vi "STS_spectroscopy_V2.vi"(6 "Internal use":string, 7 "Grid param":T1 {"height (m)" format="%#_6p"; "width (m)" format="%#_6p"; "center Y (m)" format="%#_6p"; "center X (m)" format="%#_6p"}, 8 "Error in (no error)":errorcluster, 9 "Points Y/Index Y":i32, 10 "Points X/Index X":i32, 11 "Method":enum16{"init", "run", "end"}(ring)=enum."end") -> (0 "Error out":errorcluster)   [LabVIEW 2014]
doc: "Example of a measurement VI to be used in the \"Experiments on a Grid\" tool as external VI.\n\nThis example measure the topography and spectroscopy data. The spectroscopy measurements are taken on a subgrid. The data are saved to a sxm and a binary file.\n\n- Nanonis Programming Interface -"
uses:
  <userlib>/Nanonis Prog Interface V5/Scan/Grid/LinePatternGet.vi
  <userlib>/Nanonis Prog Interface V5/Scan/Grid/GridPatternGet.vi
  <userlib>/Nanonis Prog Interface V5/Scan/Grid/CloudPatternGet.vi
  <userlib>/Nanonis Prog Interface V5/Nanonis Prog Interface.lvlib
panel:
  in  "Ramp Bias On/Off":bool
  out "Status 2":string="finishing"
  in  "Lockin delay [ms]":u32
  in  "Z Controller ON/OFF":bool
  in  "type":u16(ring)=1 items=["Line", "Grid", "Cloud"]
  in  "Lockin ON/OFF":bool
  in  "Correct Drift":bool=TRUE
  in  "Email when finished":string="cornelius.krull@monash.edu, dhaneesh.gopalakrishnan@monash.edu"
  in  "STS z offset":dbl format="%#_6p"
  out "ETA":timestamp=timestamp(3582621546.85837 s since 1904-01-01)
  out "remaining":dbl=19834.093046092985 format="%<%H:%M:%S>t"
  out "Progress":u8(slide)=5 scale=0.0..100.0 scale format="%#.1g"
  out "total Points":i32=576
  in  "preSTS delay [ms]":u32=3
  in  "STS Bias":dbl=-3.4 format="%#_6p"
  in  "Move Bias":dbl=-3.4 format="%#_6p"
  in  "Move Current":dbl=5e-11 format="%#_6p"
  in  "Imaging Bias":dbl=-3.4 format="%#_6p"
  in  "max applied Drift Correction":i32=20 min=1 max=100 step=1 format="%.0p"
  in  "Correlate":u16(ring) items=["first Frame", "successive Frames"]
  out "Topo Images taken":i32
  in  "Increment":i32=40
  in  "Threshold":i32=2 min=1 step=1
  in  "tip Speed (m/s)":sgl=1e-08 format="%.2p"
  out "X drift":i32
  out "Y drift":i32
  out "Last Drift detected":i32
  in  "MaxImagesBack":i32=2
  in  "Channel index (0-23)":u8(ring) items=["Current"=0, "Z (m)"=14]
  in  "File name":string="DCA_cluster_STS_Grid"
  in  "STS Current":dbl=5e-11 format="%#_6p"
  in  "Imaging Current":dbl=5e-11 format="%#_6p"
  in  "zdrift \nDuration (s)":dbl
  in  "Correct z drift":bool
  out "Status":string="finishing"
  in  "Drift correction Pixels":i32=256 caption="Topo Pixels"
  out "Y Offset":dbl format="%#_6p"
  out "X Offset":dbl format="%#_6p"
  out "Points taken":dbl=30.0
  in  "Drift Correction every":i32=40
  in  "Y subgrid spacing":u16=1
  in  "X subgrid spacing":u16=1
  # "GRID points"
  # "Increase this if no Drift was detected for \na certain number of images"
  # "%"
  # "time (HH:MM:SS)"
  # "images back"
  # "% of image size"
  # "<--Z Cont. Needs to be off"
  # "RUN smart tilt before starting the GRID"
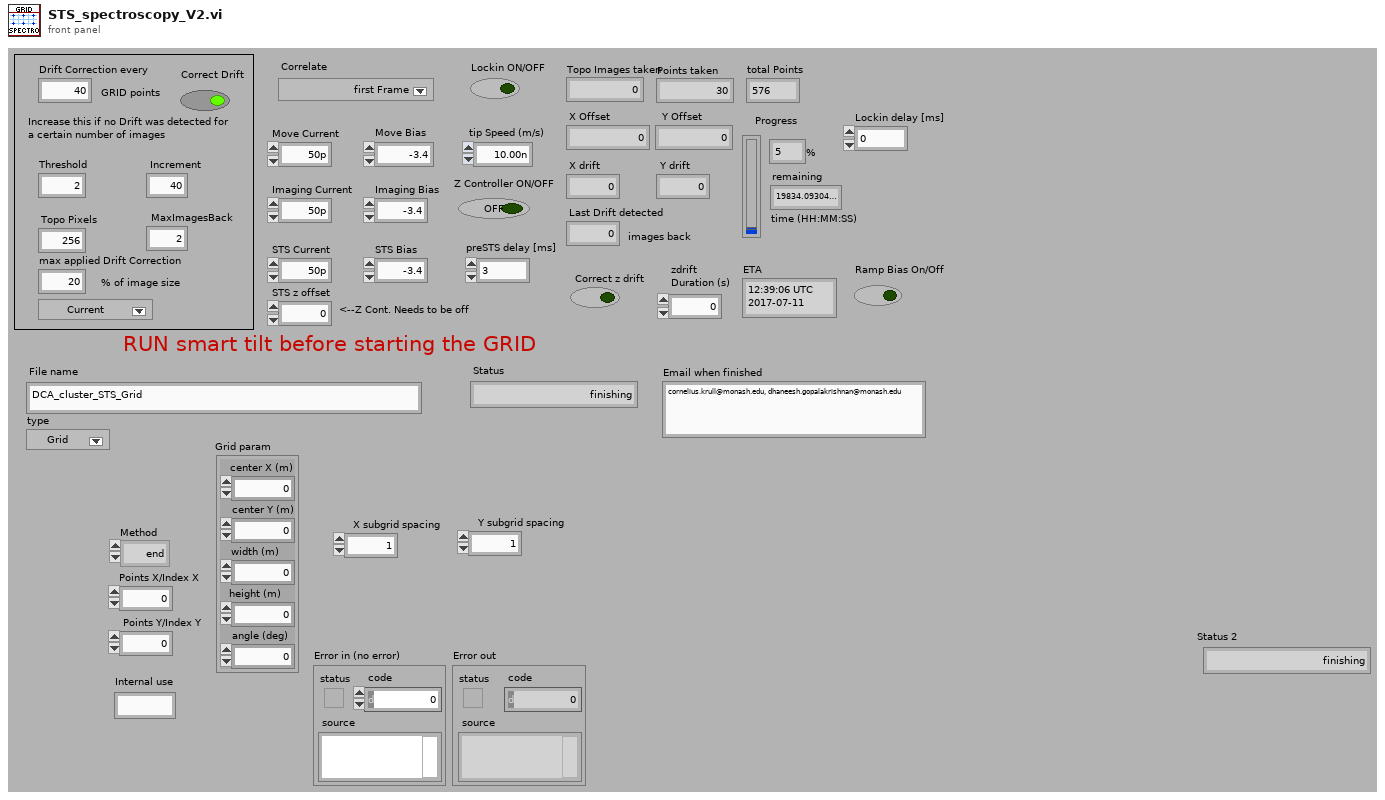
[diagram p1: front panel]
types:
  T1 = cluster{"center X (m)":sgl, "center Y (m)":sgl, "width (m)":sgl, "height (m)":sgl, "angle (deg)":sgl}
  T2 = cluster{"Drift correction Pixels":i32, "Imaging Current":dbl, "STS Current":dbl, "MaxImagesBack":i32, "tip Speed (m/s)":sgl, "Threshold":i32, "Increment":i32, "Correlate":u16, "max applied Drift Correction":i32, "Imaging Bias":dbl, "Move Current":dbl, "Move Bias":dbl, "STS Bias":dbl, "preSTS delay [ms]":u32, "STS z offset":dbl, "Correct Drift":bool, "Lockin ON/OFF":bool}
  T3 = cluster{"center X":sgl, "center Y":sgl, "angle":sgl, "width":sgl, "height":sgl, "# pixels":i32, "# lines":i32}
  T4 = cluster{"Name":string, "Calibration":sgl, "Offset":sgl, "Channel index":i32}[]
  T5 = cluster{"up/down":bool, "time/line":sgl, "start time":timestamp, "end time":timestamp}
  T6 = cluster{"Z averaging time (s)":sgl, "Z offset (m)":sgl, "Initial settling time (s)":sgl}
  T7 = cluster{"Max. slew rate (V/s)":sgl, "Settling time (s)":sgl, "Integration time (s)":sgl}
  T8 = cluster{"End settling time (s)":sgl, "Z control time (s)":sgl}
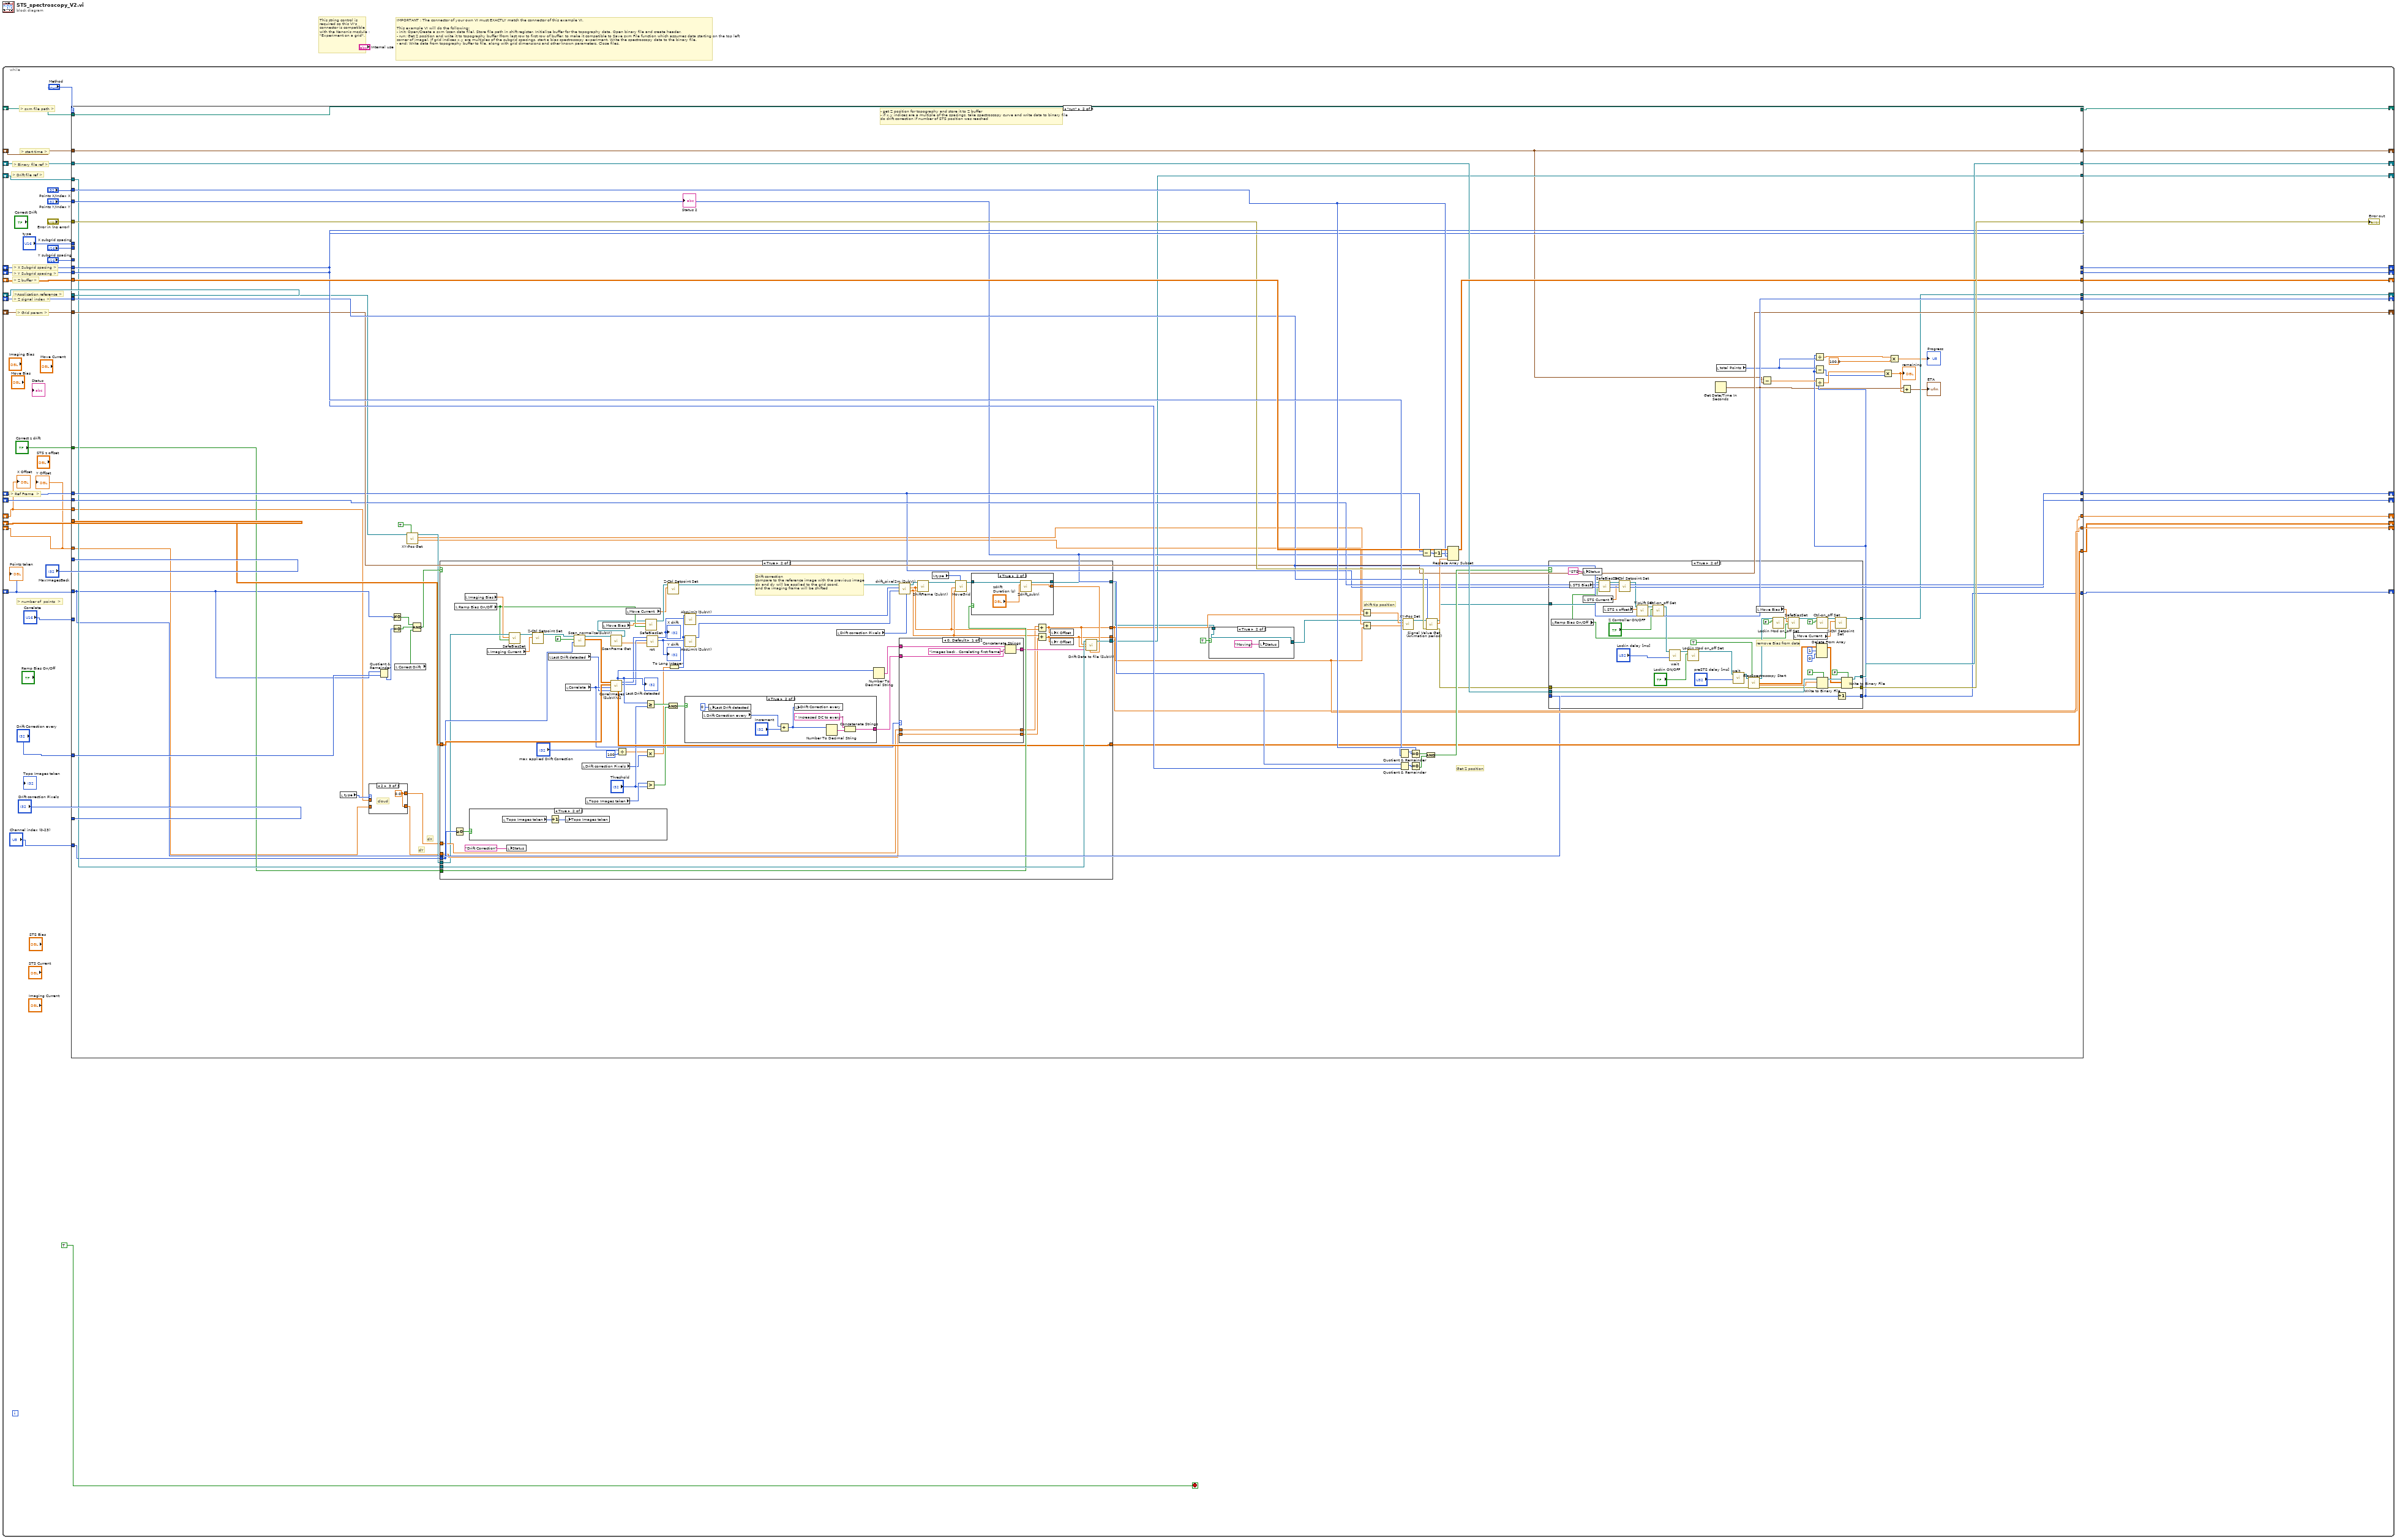
[diagram p0: block diagram]
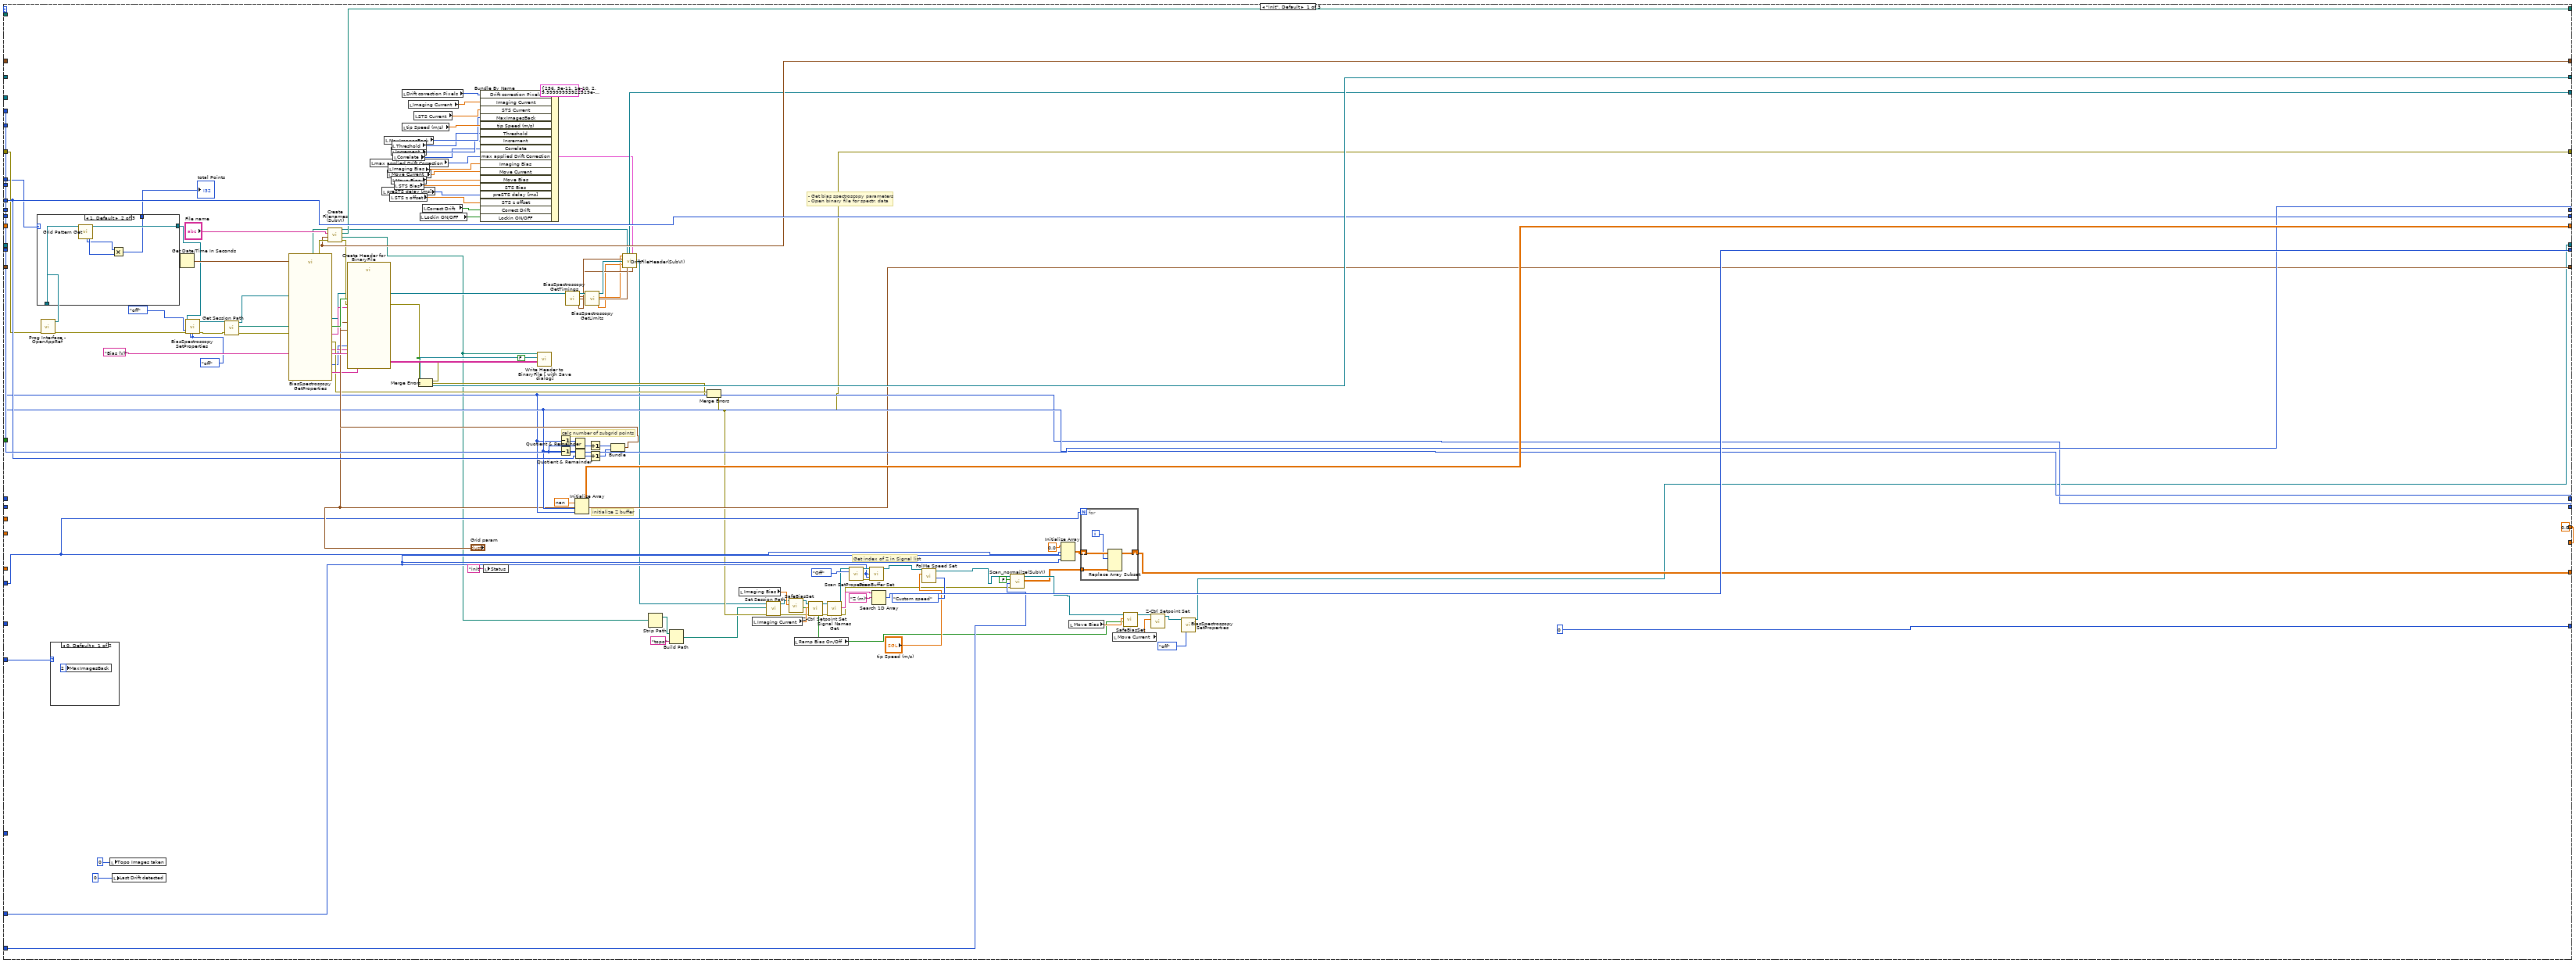
[diagram p2: hidden frame]
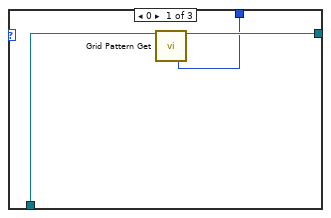
[diagram p3: hidden frame]
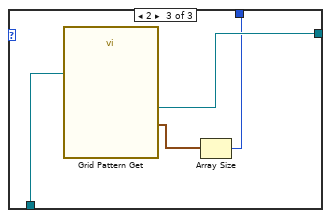
[diagram p4: hidden frame]
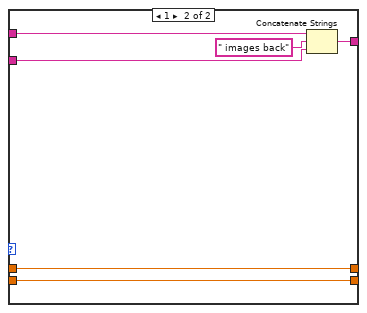
[diagram p10: hidden frame]
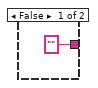
[diagram p12: hidden frame]
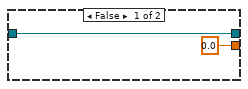
[diagram p13: hidden frame]
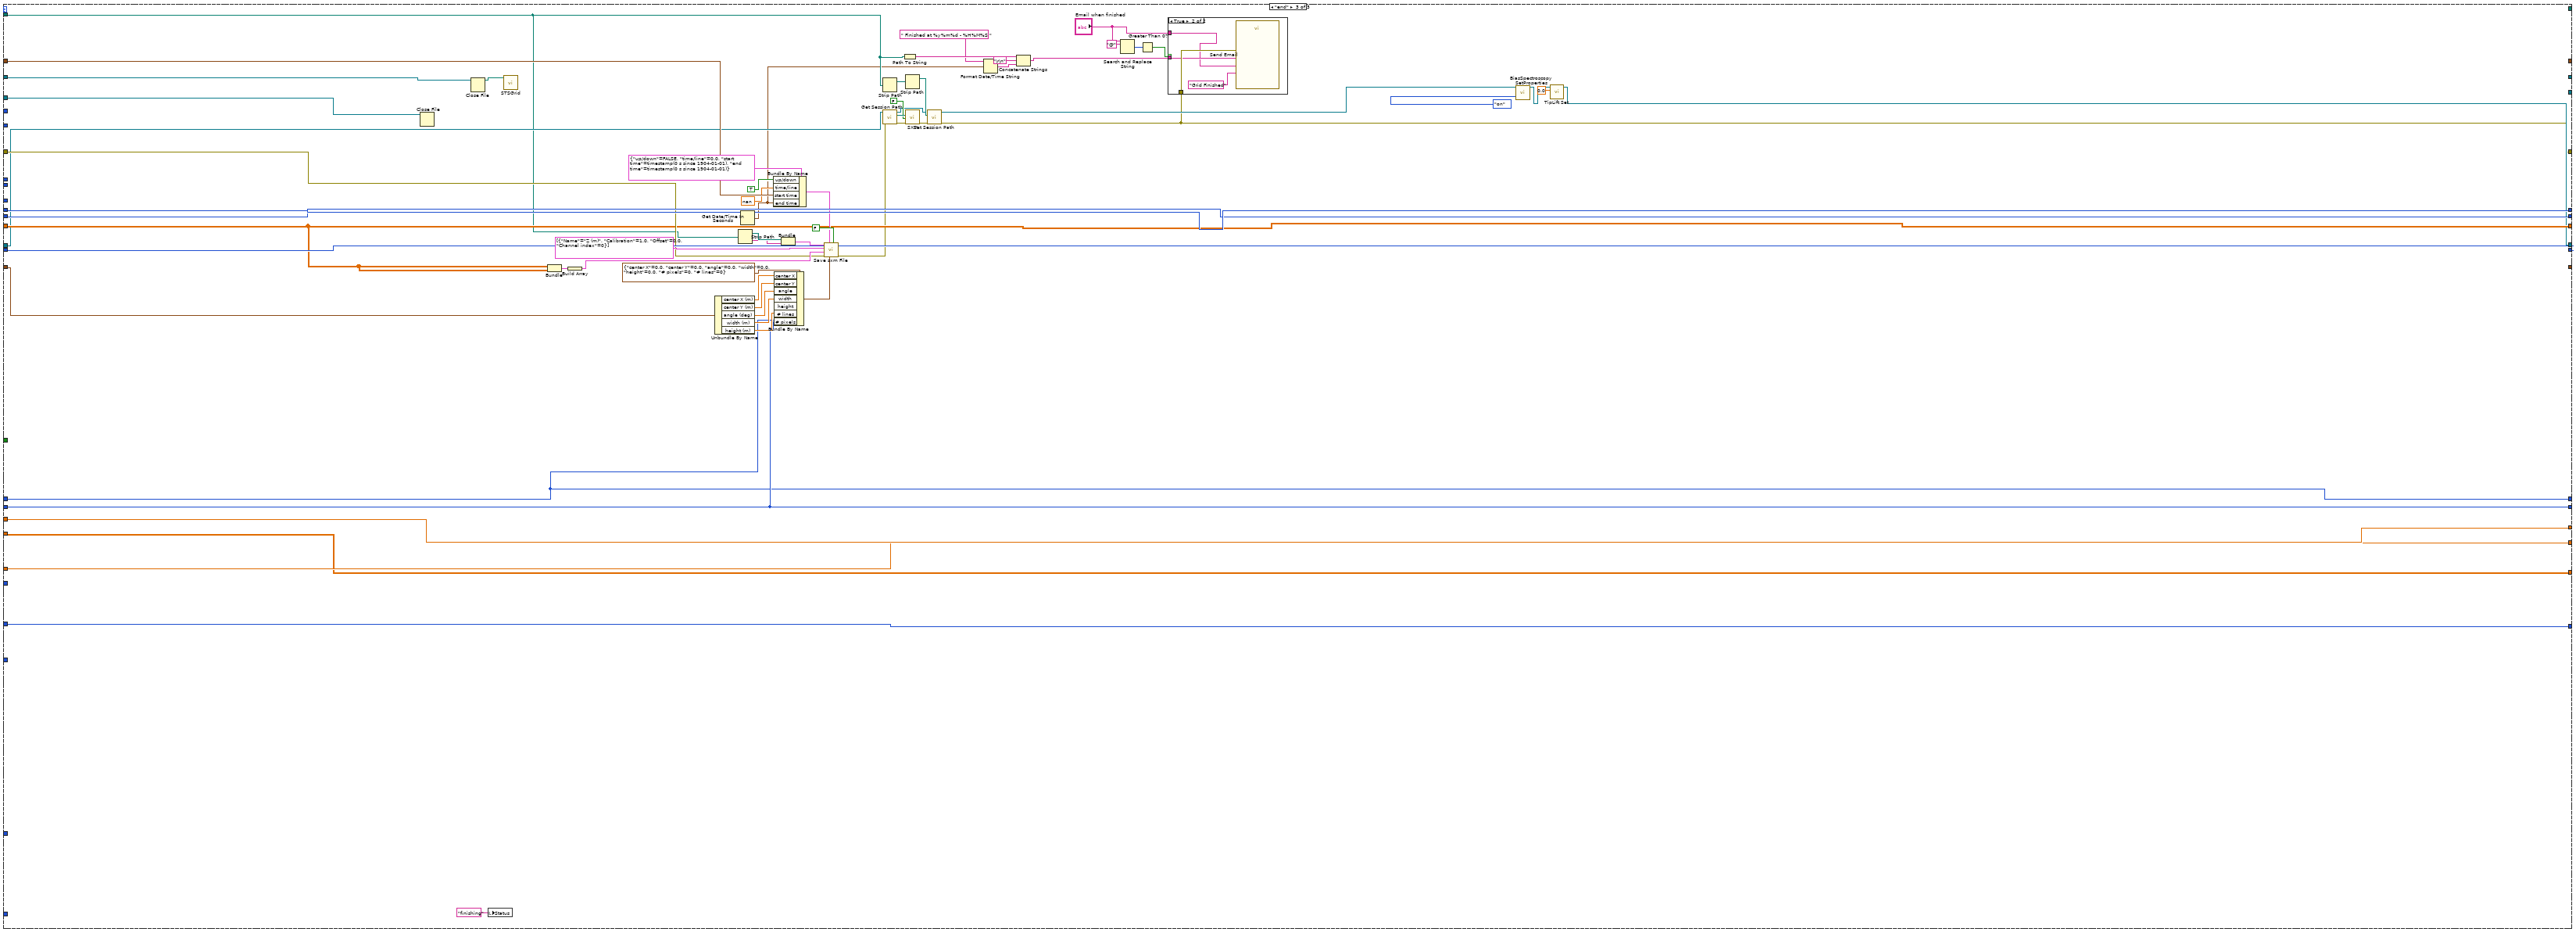
[diagram p15: hidden frame]
diagram:
  # "This string control is required so this VI's connector is compatible with the Nanonis module : \"Experiment on a grid\"."
  # "IMPORTANT : The connector of your own VI must EXACTLY match the connector of this example VI.\n\nThis example VI will do the following:\n- init: Open/Create a sxm (scan data file). Store file path in shift register. Initialize buffer for the topography data. Open binary file and create header.\n- run: Get Z position and write it to topography buffer (from last row to first row of buffer, to make it compatible to Save sxm File function which assumes data starting on the top left corner of image). If grid indices x,y are multiples of the subgrid spacings, start a bias spectroscopy experiment. Write the spectroscopy data to the binary file.\n- end: Write data from topography buffer to file, along with grid dimensions and other known parameters. Close files."
  n1 = while {
    shift-right: [w22] -> _
    shift-left: _ -> [w45]
    shift-right: [w40] -> _
    shift-left: _ -> [w39]
    shift-right: [w37] -> _
    shift-left: _ -> [w38]
    shift-right: [w36] -> _
    shift-left: _ -> [w35]
    shift-right: [w29] -> _
    shift-left: _ -> [w31]
    shift-right: [w30] -> _
    shift-left: _ -> [w32]
    shift-right: [w28] -> _
    shift-left: _ -> [w27]
    shift-right: [w26] -> _
    shift-left: _ -> [w25]
    shift-right: [w24] -> _
    shift-left: _ -> [w23]
    shift-right: [w21] -> _
    shift-left: _ -> [w20]
    shift-right: [w19] -> _
    shift-left: _ -> [w18]
    shift-right: [w17] -> _
    shift-left: _ -> [w10]
    shift-right: [w16] -> _
    shift-left: _ -> [w9]
    shift-right: [w15] -> _
    shift-left: _ -> [w12]
    shift-right: [w14] -> _
    shift-left: _ -> [w11]
    shift-right: [w7] -> _
    shift-left: _ -> [w6]
    stop <- TRUE stop-if-true
    # "> Drift file ref >"
    # "> number of  points  >"
    # "> Ref Frame  >"
    # "> Grid param >"
    # "> start time >"
    # ">Application reference >"
    # "> Y Subgrid spacing >"
    # "> X Subgrid spacing >"
    # "> Z signal index >"
    # "> Binary file ref >"
    # "> Z buffer >"
    # "> sxm file path >"
    n2 = case shown="\"run\"" "Method" {
      tunnel: [w128 w252 _] -> w22
      tunnel: w45 -> [_ w252 w421]
      tunnel: "Error in (no error)" -> [w130 w238 w448]
      tunnel: [w53 w251 w402] -> w43
      tunnel: "Points X/Index X" -> [w142 w246 _]
      tunnel: "Points Y/Index Y" -> [w143 w231 _]
      tunnel: [w166 w249 w437] -> w40
      tunnel: w39 -> [_ w250 w437]
      tunnel: w38 -> [_ w248 w430]
      tunnel: [w158 w247 _] -> w37
      tunnel: [w156 w236 w462] -> w36
      tunnel: w35 -> [_ w236 w462]
      tunnel: "X subgrid spacing" -> [w155 _ _]
      tunnel: "Y subgrid spacing" -> [w154 _ _]
      tunnel: w32 -> [_ w240 w461]
      tunnel: w31 -> [_ w239 w460]
      tunnel: [w155 w240 w461] -> w30
      tunnel: [w154 w239 w460] -> w29
      tunnel: [w92 w225 w408] -> w28
      tunnel: w27 -> [_ w209 w425]
      tunnel: ["Grid param" w234 _] -> w26
      tunnel: w25 -> [_ w234 w447]
      tunnel: [w127 w200 _] -> w24
      tunnel: w23 -> [_ w200 w455]
      tunnel: [w143 w232 w438] -> w21
      tunnel: w20 -> [_ w232 w438]
      tunnel: [w142 w233 w439] -> w19
      tunnel: w18 -> [_ w233 w439]
      tunnel: [w139 w215 w436] -> w17
      tunnel: [w139 w220 w434] -> w16
      tunnel: [w123 w214 w431] -> w15
      tunnel: [0 w198 w435] -> w14
      tunnel: w11 -> [_ w212 w435]
      tunnel: "Drift Correction every" -> [_ w227 _]
      tunnel: w12 -> [_ w219 w431]
      tunnel: w10 -> [_ w187 w436]
      tunnel: w9 -> [_ w185 w434]
      tunnel: "Drift correction Pixels" -> [w122 _ _]
      tunnel: [w87 w217 _] -> w7
      tunnel: w6 -> [_ w218 w432]
      tunnel: "Correct z drift" -> [_ w216 _]
      tunnel: "Channel index (0-23)" -> [w61 w213 _]
      tunnel: "MaxImagesBack" -> [w121 _ _]
      tunnel: "Correlate" -> [w103 _ _]
      tunnel: "type" -> [w55 _ _]
      frame "init", Default {
        w89 = enum16{"no change", "on", "off"}."off" ("Save dialog")
        w139 = 0.0
        # "- Get bias spectroscopy parameters\n- Open binary file for spectr. data"
        # "initialize Z buffer"
        # "calc number of subgrid points"
        # "Get index of Z in Signal list"
        n3 = call <userlib>:"Prog Interface - OpenAppRef.vi"("Error in (no error)"=w130) -> ("Error out"=w109:errorcluster, "Application reference"=w94:refnum<vi>)  [unwired: 5 in]
        n4 = case shown="1, Default" w55 {
          tunnel: w94 -> [w169 w174 w178]
          tunnel: [w168 w173 w177] -> w93
          tunnel: [w167 w170 w175] -> w54
          frame 0 {
            n5 = call-poly <userlib>:"Grid Pattern Get.vi"("Application ref in"=w169) -> ("Points"=w167:i32, "Application ref out"=w168:refnum<vi>)  [unwired: 12 in, 5 out]
          }
          frame 1, Default {
            n6 = call-poly <userlib>:"Grid Pattern Get.vi"("Application ref in"=w174) -> ("Points Y"=w171:i32, "Points X"=w172:i32, "Application ref out"=w173:refnum<vi>)  [unwired: 10 in, 6 out]
            n7 = Multiply(x=w171, y=w172) -> (x*y=w170:i32)
          }
          frame 2 {
            n8 = call-poly <userlib>:"Grid Pattern Get.vi"("Application ref in"=w178) -> ("Application ref out"=w177:refnum<vi>, "Cloud data"=w176:cluster{"X":sgl, "Y":sgl}[])  [unwired: 16 in, 1 out]
            n9 = Array Size(array=w176) -> (size(s)=w175:i32)
          }
        }
        "total Points" <- w54
        n10 = case shown="0, Default" w103 {
          frame 0, Default {
            n11 = local write "MaxImagesBack"(2 ("StepsBack")) -> ()
          }
          frame 1 {
          }
        }
        n12 = local write "Topo Images taken"(0 ("Images taken")) -> ()
        n13 = local write "Last Drift detected"(0 ("Last Drift detected")) -> ()
        n14 = Get Date/Time In Seconds() -> (seconds since 1Jan1904=w127:timestamp)
        n15 = call <userlib>:"BiasSpectroscopy SetProperties.vi"("Application ref in"=w93, "Autosave (no change)"=enum16{"no change", "on", "off"}."off", "Error in (no error)"=w109, "Z-Controller hold (no change)"=w89, "Save dialog"=w89) -> ("Application ref out"=w106:refnum<vi>, "Error out"=w105:errorcluster)  [unwired: 9 in]
        n16 = call <userlib>:"Get Session Path.vi"("error in (no error)"=w105, "Application ref in"=w106) -> ("error out"=w129:errorcluster, "Session path"=w113:path, "Application ref out"=w107:refnum<vi>)  [unwired: 7 in]
        n17 = call <userlib>:"BiasSpectroscopy GetProperties.vi"("Application ref in"=w107) -> ("Backward sweep"=w162:bool, "Application ref out"=w116:refnum<vi>, "Number of points"=w145:i32, "Channels"=w144:string[], "Parameters"=w160:string[], "Fixed parameters"=w147:string[], "Error out"=w159:errorcluster)  [unwired: 6 in, 2 out]
        n18 = call "Create Filenames (SubVI).vi"("error in (no error)"=w129, "seconds since 1Jan1904"=w127, "File name"="File name", "Session path"=w113) -> ("error out"=w117:errorcluster, "binFilePath"=w110:path, "topoFilePath"=w128:path, "Drift File out"=w88:refnum<file>)  [unwired: 4 in]
        n19 = local read "max applied Drift Correction"() -> (w69:i32)
        n20 = local read "preSTS delay [ms]"() -> (w64:u32)
        n21 = local read "MaxImagesBack"() -> (w73:i32)
        n22 = local read "Move Current"() -> (w67:dbl)
        n23 = local read "Imaging Bias"() -> (w68:dbl)
        n24 = local read "STS z offset"() -> (w63:dbl)
        n25 = local read "Increment"() -> (w71:i32)
        n26 = local read "Move Bias"() -> (w66:dbl)
        n27 = local read "Threshold"() -> (w72:i32)
        n28 = local read "Correlate"() -> (w70:u16)
        n29 = local read "STS Bias"() -> (w65:dbl)
        n30 = local read "Drift correction Pixels"() -> (w78:i32)
        n31 = local read "tip Speed (m/s)"() -> (w75:sgl)
        n32 = local read "Imaging Current"() -> (w77:dbl)
        n33 = local read "STS Current"() -> (w76:dbl)
        n34 = local read "Lockin ON/OFF"() -> (w74:bool)
        n35 = local read "Correct Drift"() -> (w62:bool)
        n36 = Bundle By Name(cluster=T2 {"Drift correction Pixels"=256, "Imaging Current"=5e-11, "STS Current"=1e-10, "MaxImagesBack"=2, "tip Speed (m/s)"=1e-08, "Threshold"=2, "Increment"=64, "Correlate"=0, "max applied Drift Correction"=20, "Imaging Bias"=-0.02, "Move Current"=1.5e-11, "Move Bias"=-0.02, "STS Bias"=0.1, "preSTS delay [ms]"=1000, "STS z offset"=-1.7e-10, "Correct Drift"=TRUE, "Lockin ON/OFF"=TRUE} ("Drift Correction"), "Drift correction Pixels"=w78, "Imaging Current"=w77, "STS Current"=w76, "MaxImagesBack"=w73, "tip Speed (m/s)"=w75, "Threshold"=w72, "Increment"=w71, "Correlate"=w70, "max applied Drift Correction"=w69, "Imaging Bias"=w68, "Move Current"=w67, "Move Bias"=w66, "STS Bias"=w65, "preSTS delay [ms]"=w64, "STS z offset"=w63, "Correct Drift"=w62, "Lockin ON/OFF"=w74) -> (w80:T2)
        n37 = local write "Status"("init" ("Status")) -> ()
        n38 = Decrement(x=w142) -> (x-1=w153:i32)
        n39 = Decrement(x=w143) -> (x-1=w152:i32)
        n40 = call <userlib>:"BiasSpectroscopy GetTimings.vi"("Application ref in"=w116) -> ("Application ref out"=w120:refnum<vi>, "Initialization"=w83:T6, "Sweep Timing"=w84:T7, "End of Sweep"=w85:T8)  [unwired: 10 in, 1 out]
        n41 = Quotient & Remainder(x=w153, y=w155) -> (floor(x/y)=w151:i32)  [unwired: 1 out]
        n42 = Quotient & Remainder(x=w152, y=w154) -> (floor(x/y)=w150:i32)  [unwired: 1 out]
        n43 = Initialize Array(sgl nan ("element"), w143, w142) -> (w166:sgl[][])
        n44 = call <userlib>:"BiasSpectroscopy GetLimits.vi"("Application ref in"=w120) -> ("End value (V)"=w81:sgl, "Start value (V)"=w82:sgl, "Application ref out"=w86:refnum<vi>)  [unwired: 5 in, 1 out]
        n45 = Increment(x=w151) -> (x+1=w149:i32)
        n46 = Increment(x=w150) -> (x+1=w148:i32)
        n47 = Bundle(w149, w148) -> (w161:cluster{i32, i32})  [unwired: 1 in]
        n48 = call <userlib>:"Create Header for BinaryFile.vi"("Grid points"=w161, "Grid param"="Grid param", "Fixed parameters"=w147, "Backward sweep"=w162, "Sweep signal"="Bias (V)" ("Sweep Signal"), "Parameters"=w160, "Channels"=w144, "Points per sweep"=w145) -> ("Header (fixed attributes)"=w164:string[][])  [unwired: 3 in]
        n49 = call <userlib>:"Write Header to BinaryFile [ with Save dialog].vi"("Fixed Attributes"=w164, "Show Dialog? (T)"=FALSE, "Filename"=w110) -> ("Error out"=w118:errorcluster, "File ref"=w158:refnum<file>)  [unwired: 5 in, 2 out]
        n50 = Merge Errors(w118, w117) -> (w119:errorcluster)
        n51 = call "DriftFileHeader(SubVI).vi"("Start value (V)"=w82, "Byte Stream File in"=w88, "Drift Correction"=w80, "End of Sweep"=w85, "Application ref in"=w86, "End value (V)"=w81, "Sweep Timing"=w84, "Initialization"=w83) -> ("Byte Stream File out"=w87:refnum<file>, "Application ref out"=w50:refnum<vi>)  [unwired: 6 in]
        n52 = Strip Path(path=w110) -> (stripped path=w112:path)  [unwired: 1 out]
        n53 = Build Path(base path=w112, name or relative path="topo") -> (appended path=w52:path)
        n54 = Merge Errors(w159, w119) -> (w53:errorcluster)
        n55 = local read "Imaging Bias"() -> (w96:dbl)
        n56 = local read "Imaging Current"() -> (w95:dbl)
        n57 = call <userlib>:"Set Session Path.vi"("error in (no error)"=w53, "Session Folder"=w52, "Application ref in"=w50) -> ("error out"=w51:errorcluster, "Application ref out"=w49:refnum<vi>)  [unwired: 7 in]
        n58 = local read "Ramp Bias On/Off"() -> (w48:bool)
        n59 = call "SafeBiasSet.vi"("Application ref in"=w49, "Bias (V)"=w96, "Ramp"=w48) -> ("Application ref out"=w99:refnum<vi>)  [unwired: 6 in, 1 out]
        n60 = call <userlib>:"Z-Ctrl Setpoint Set.vi"("error in (no error)"=w51, "Z Controller setpoint"=w95, "Application ref in"=w99) -> ("error out"=w131:errorcluster, "Application ref out"=w132:refnum<vi>)  [unwired: 7 in]
        n61 = call <userlib>:"Signal Names Get.vi"("error in (no error)"=w131, "Application ref in"=w132) -> ("error out"=w58:errorcluster, "Signals Names"=w146:string[], "Application ref out"=w135:refnum<vi>)  [unwired: 5 in]
        n62 = call <userlib>:"Scan SetProperties.vi"("Application ref in"=w135, "Continuous scan"=enum16{"No change", "On", "Off"}."Off") -> ("Application ref out"=w137:refnum<vi>, "Error out"=w136:errorcluster)  [unwired: 12 in]
        n63 = call <userlib>:"ScanBuffer Set.vi"("Application ref in"=w137, "Pixels"=w122, "Lines"=w122, "error in (no error)"=w136) -> ("Application ref out"=w101:refnum<vi>)  [unwired: 10 in, 1 out]
        n64 = Search 1D Array(1D array=w146, element="Z (m)") -> (index of element=w156:i32)  [unwired: 1 in]
        n65 = call <userlib>:"FolMe Speed Set.vi"("Speed Setting (Custom)"=enum32{"Scan speed", "Custom speed"}."Custom speed", "Speed (m/s)"="tip Speed (m/s)", "Application ref in"=w101) -> ("Application ref out"=w60:refnum<vi>)  [unwired: 5 in, 1 out]
        n66 = call "Scan_normailze(SubVI).vi"("error in (no error)"=w58, "Channel index (0-23)"=w61, "Normalization"=FALSE ("Boolean"), "Application in"=w60) -> ("Array"=w57:dbl[][], "Application out"=w59:refnum<vi>)  [unwired: 5 in, 1 out]
        n67 = Initialize Array(0.0 ("element"), w121, w122, w122) -> (w124:dbl[][][])
        n68 = local read "Move Bias"() -> (w98:dbl)
        n69 = for {
          N: w121 -> [_]
          tunnel: w57 -> [w182]
          shift-right: [w181] -> w123
          shift-left: w124 -> [w183]
          i -> [w180]
          n70 = Replace Array Subset(array=w183, new element=w182, index (dim 0)=w180) -> (w181:dbl[][][])  [unwired: 2 in]
        }
        n71 = local read "Move Current"() -> (w97:dbl)
        n72 = call "SafeBiasSet.vi"("Application ref in"=w59, "Bias (V)"=w98, "Ramp"=w48) -> ("Application ref out"=w100:refnum<vi>)  [unwired: 6 in, 1 out]
        n73 = call <userlib>:"Z-Ctrl Setpoint Set.vi"("Z Controller setpoint"=w97, "Application ref in"=w100) -> ("Application ref out"=w91:refnum<vi>)  [unwired: 8 in, 1 out]
        n74 = call <userlib>:"BiasSpectroscopy SetProperties.vi"("Application ref in"=w91, "Z-Controller hold (no change)"=enum16{"no change", "on", "off"}."off") -> ("Application ref out"=w92:refnum<vi>)  [unwired: 12 in, 1 out]
      }
      frame "run" {
        # "dX"
        # "dY"
        # "shift tip position"
        # "Get Z position"
        # "- get Z position for topography and store it to Z buffer\n- if x,y indices are a multiple of the spacings, take spectroscopy curve and write data to binary file\ndo drift correction if number of STS position was reached"
        n75 = local read "type"() -> (w188:u16)
        n76 = case shown="2" w188 {
          tunnel: w187 -> [w253 w256 _]
          tunnel: [w253 w256 w257] -> w186
          tunnel: [w254 w255 w257] -> w184
          tunnel: w185 -> [w254 w255 _]
          frame 0, Default {
            # "grid"
          }
          frame 1 {
            # "line"
          }
          frame 2 {
            w257 = 0.0
            # "cloud"
          }
        }
        n77 = Quotient & Remainder(x=w212, y=w227) -> (x-y*floor(x/y)=w228:i32)  [unwired: 1 out]
        n78 = Not Equal To 0?(x=w212) -> (x != 0?=w210:bool)
        n79 = Equal To 0?(x=w228) -> (x = 0?=w226:bool)
        n80 = local read "Correct Drift"() -> (w192:bool)
        n81 = call <userlib>:"XY-Pos Get.vi"("Wait for newest data (F=False)"=TRUE, "Application ref in"=w209) -> ("Y (m)"=w205:sgl, "X (m)"=w206:sgl, "Application ref out"=w208:refnum<vi>)  [unwired: 5 in, 1 out]
        n82 = Compound Arithmetic op=AND(w210, w226, w192) -> (w211:bool)
        n83 = case shown="True" w211 {
          tunnel: w208 -> [w265 w282]
          tunnel: [w265 w322] -> w191
          tunnel: w219 -> [w264 w317]
          tunnel: [w262 w320] -> w215
          tunnel: [w261 w319] -> w220
          tunnel: w186 -> [w262 w296]
          tunnel: w184 -> [w261 w294]
          tunnel: [w264 w313] -> w214
          tunnel: w218 -> [w263 w325]
          tunnel: [w263 w324] -> w217
          tunnel: w216 -> [_ w321]
          tunnel: w213 -> [_ w300]
          frame False {
          }
          frame True {
            # "Drift correction \ncompare to the reference image with the previous image \ndx and dy will be applied to the grid coord, \nand the imaging frame will be shifted"
            n84 = Greater Or Equal To 0?(x=w300) -> (x >= 0?=w299:bool)
            n85 = local read "Ramp Bias On/Off"() -> (w273:bool)
            n86 = local read "Imaging Bias"() -> (w280:dbl)
            n87 = case shown="True" w299 {
              frame False {
              }
              frame True {
                n88 = local read "Topo Images taken"() -> (w340:i32)
                n89 = Increment(x=w340) -> (x+1=w339:i32)
                n90 = local write "Topo Images taken"(w339) -> ()
              }
            }
            n91 = local read "Imaging Current"() -> (w279:dbl)
            n92 = local write "Status"("Drift Correction" ("Status")) -> ()
            n93 = call "SafeBiasSet.vi"("Application ref in"=w282, "Bias (V)"=w280, "Ramp"=w273) -> ("Application ref out"=w281:refnum<vi>)  [unwired: 6 in, 1 out]
            n94 = call <userlib>:"Z-Ctrl Setpoint Set.vi"("Z Controller setpoint"=w279, "Application ref in"=w281) -> ("Application ref out"=w318:refnum<vi>)  [unwired: 8 in, 1 out]
            n95 = local read "Last Drift detected"() -> (w291:i32)
            n96 = local read "Correlate"() -> (w297:u16)
            n97 = call "Scan_normailze(SubVI).vi"("Channel index (0-23)"=w300, "Normalization"=FALSE ("Boolean"), "Application in"=w318) -> ("Array"=w314:dbl[][], "Application out"=w270:refnum<vi>)  [unwired: 6 in, 1 out]
            n98 = local read "Drift correction Pixels"() -> (w288:i32)
            n99 = local read "Topo Images taken"() -> (w302:i32)
            n100 = local read "Move Bias"() -> (w277:dbl)
            n101 = call <userlib>:"ScanFrame Get.vi"("Application ref in"=w270) -> ("Application ref out"=w266:refnum<vi>, "Angle (deg)"=w269:sgl)  [unwired: 10 in, 3 out]
            n102 = call "CorrelImages (SubVI)v2.vi"("last drift detected"=w291, "Correlate"=w297, "Ref Array"=w317, "New Image"=w314) -> ("Y drift"=w271:i32, "X drift"=w272:i32, "Ref Array out"=w313:dbl[][][], "Queue Steps"=w298:i32)  [unwired: 4 in]
            "Last Drift detected" <- w298
            n103 = Divide(x="max applied Drift Correction", y=100) -> (x/y=w287:dbl)
            n104 = local read "Move Current"() -> (w276:dbl)
            n105 = Greater Or Equal?(x=w298, y="Threshold") -> (x >= y?=w304:bool)
            n106 = Multiply(x=w287, y=w288) -> (x*y=w289:dbl)
            n107 = Greater?(x=w302, y="Threshold") -> (0:w301:bool)
            n108 = call "SafeBiasSet.vi"("Application ref in"=w266, "Bias (V)"=w277, "Ramp"=w273) -> ("Application ref out"=w278:refnum<vi>)  [unwired: 6 in, 1 out]
            n109 = call "rot.vi"("angle"=w269, "y"=w271, "x"=w272) -> ("y'"=w267:i32, "x'"=w268:i32)  [unwired: 7 in]
            "X drift" <- w268
            "Y drift" <- w267
            n110 = And(x=w304, y=w301) -> (x .and. y?=w303:bool)
            n111 = call <userlib>:"Z-Ctrl Setpoint Set.vi"("Z Controller setpoint"=w276, "Application ref in"=w278) -> ("Application ref out"=w309:refnum<vi>)  [unwired: 8 in, 1 out]
            n112 = To Long Integer(number=w289) -> (32bit integer=w283:i32)
            n113 = call "AbsLimit (SubVI).vi"("in"=w268, "Abslimt"=w283) -> ("Numeric out"=w285:i32)  [unwired: 9 in]
            n114 = call "AbsLimit (SubVI).vi"("in"=w267, "Abslimt"=w283) -> ("Numeric out"=w284:i32)  [unwired: 9 in]
            n115 = case shown="True" w303 {
              tunnel: ["" w344] -> w305
              frame False {
              }
              frame True {
                n116 = local read "Drift Correction every"() -> (w343:i32)
                n117 = local write "Last Drift detected"(0 ("Last Drift detected")) -> ()
                n118 = Add(x=w343, y="Increment") -> (x+y=w347:i32)
                n119 = local write "Drift Correction every"(w347) -> ()
                n120 = Number To Decimal String(number=w347) -> (decimal integer string=w346:string)  [unwired: 1 in]
                n121 = Concatenate Strings(" Increased DC to every " ("string"), w346) -> (w344:string)
              }
            }
            n122 = local read "Drift correction Pixels"() -> (w310:i32)
            n123 = Number To Decimal String(number=w298) -> (decimal integer string=w316:string)  [unwired: 1 in]
            n124 = call "drift_pixel2m (SubVI).vi"("Application in"=w309, "X drift"=w285, "Y drift"=w284, "Drift correction Pixels"=w310) -> ("Application out"=w308:refnum<vi>, "x drift"=w306:sgl, "y drift"=w307:sgl)  [unwired: 2 in, 1 out]
            n125 = case shown="0, Default" w297 {
              tunnel: w316 -> [w327 w338]
              tunnel: [w332 w337] -> w315
              tunnel: w305 -> [w330 w335]
              tunnel: w296 -> [w328 w334]
              tunnel: [w328 w334] -> w295
              tunnel: w294 -> [w329 w333]
              tunnel: [w329 w333] -> w293
              frame 0, Default {
                n126 = Concatenate Strings(w327, "images back , Correlating first frame " ("string"), w330) -> (w332:string)
              }
              frame 1 {
                n127 = Concatenate Strings(w338, " images back" ("string"), w335) -> (w337:string)
              }
            }
            n128 = call "ShiftFrame (SubVI).vi"("Y shift"=w307, "X shift"=w306, "Application in"=w308) -> ("Application out"=w312:refnum<vi>)  [unwired: 8 in]
            n129 = local read "type"() -> (w274:u16)
            n130 = call "MoveGrid.vi"("type"=w274, "y"=w307, "x"=w306, "Application ref in"=w312) -> ("Application ref out"=w311:refnum<vi>)  [unwired: 6 in, 1 out]
            n131 = case shown="True" w321 {
              tunnel: [0.0 ("z drift") w354] -> w323
              tunnel: w311 -> [w349 w353]
              tunnel: [w349 w352] -> w322
              frame False {
              }
              frame True {
                n132 = call "Zdrift_subVi.vi"("Duration"="zdrift \nDuration (s)", "Application in"=w353) -> ("z drift"=w354:dbl, "Application out"=w352:refnum<vi>)  [unwired: 7 in, 1 out]
              }
            }
            n133 = Add(x=w295, y=w306) -> (x+y=w320:dbl)
            n134 = Add(x=w307, y=w293) -> (x+y=w319:dbl)
            n135 = local write "X Offset"(w320) -> ()
            n136 = local write "Y Offset"(w319) -> ()
            n137 = call "Drift Data to file (SubVI).vi"("z drift"=w323, "Comment"=w315, "y Drift"=w319, "X drift"=w320, "Byte Stream File in"=w325) -> ("Byte Stream File out"=w324:refnum<file>)  [unwired: 6 in]
          }
        }
        n138 = case shown="True" TRUE {
          tunnel: [w258 w259] -> w190
          tunnel: w191 -> [w258 w259]
          frame False {
          }
          frame True {
            n139 = local write "Status"("Moving" ("Status")) -> ()
          }
        }
        n140 = Add(x=w206, y=w215) -> (x+y=w222:dbl)
        n141 = Add(x=w205, y=w220) -> (x+y=w221:dbl)
        n142 = Quotient & Remainder(x=w246, y=w240) -> (x-y*floor(x/y)=w245:i32)  [unwired: 1 out]
        n143 = Quotient & Remainder(x=w231, y=w239) -> (x-y*floor(x/y)=w244:i32)  [unwired: 1 out]
        n144 = call <userlib>:"XY-Pos Set.vi"("Y (m)"=w221, "X (m)"=w222, "Application ref in"=w190) -> ("Application ref out"=w223:refnum<vi>)  [unwired: 5 in, 1 out]
        n145 = Equal To 0?(x=w245) -> (x = 0?=w243:bool)
        n146 = Equal To 0?(x=w244) -> (x = 0?=w242:bool)
        n147 = Subtract(x=w232, y=w231) -> (x-y=w230:i32)
        n148 = And(x=w243, y=w242) -> (x .and. y?=w241:bool)
        n149 = call <userlib>:"Signal Value Get (Animation period).vi"("error in (no error)"=w238, "Signal index (0-47)"=w236, "Application ref in"=w223) -> ("error out"=w237:errorcluster, "Signal value"=w235:sgl, "Application ref out"=w224:refnum<vi>)  [unwired: 5 in]
        n150 = Decrement(x=w230) -> (x-1=w229:i32)
        n151 = Replace Array Subset(array=w250, new element=w235, index (row)=w229, index (col)=w246) -> (w249:sgl[][])
        n152 = case shown="True" w241 {
          tunnel: [w357 w387] -> w251
          tunnel: w248 -> [w358 w401]
          tunnel: [w358 w399] -> w247
          tunnel: w237 -> [w357 w398]
          tunnel: w224 -> [w356 w383]
          tunnel: [w356 w378] -> w225
          tunnel: [w355 w385] -> w198
          tunnel: w212 -> [w355 w386]
          frame False {
            # "Point indices aren't multiple of subgrid spacing\n=> no spectroscopy at this point"
          }
          frame True {
            # "remove Bias from data"
            n153 = local read "Ramp Bias On/Off"() -> (w360:bool)
            n154 = local read "STS Bias"() -> (w380:dbl)
            n155 = local write "Status"("STS" ("Status")) -> ()
            n156 = local read "STS Current"() -> (w379:dbl)
            n157 = call "SafeBiasSet.vi"("Application ref in"=w383, "Bias (V)"=w380, "Ramp"=w360) -> ("Application ref out"=w382:refnum<vi>)  [unwired: 6 in, 1 out]
            n158 = local read "STS z offset"() -> (w367:dbl)
            n159 = call <userlib>:"Z-Ctrl Setpoint Set.vi"("Z Controller setpoint"=w379, "Application ref in"=w382) -> ("Application ref out"=w375:refnum<vi>)  [unwired: 8 in, 1 out]
            n160 = call <userlib>:"TipLift Set.vi"("TipLift (m)"=w367, "Application ref in"=w375) -> ("Application ref out"=w365:refnum<vi>)  [unwired: 8 in, 1 out]
            n161 = call <userlib>:"Ctrl-on_off Set.vi"("Z Controller ON/OFF"="Z Controller ON/OFF", "Application ref in"=w365) -> ("Application ref out"=w363:refnum<vi>)  [unwired: 8 in, 1 out]
            n162 = call "wait.vi"("milliseconds to wait"="Lockin delay [ms]", "application reference in"=w363) -> ("application reference out"=w362:refnum<vi>)  [unwired: 8 in, 1 out]
            n163 = call <userlib>:"Lockin Mod on_off Set.vi"("Lockin ON/OFF"="Lockin ON/OFF", "Application ref in"=w362) -> ("Application ref out"=w359:refnum<vi>)  [unwired: 8 in, 1 out]
            n164 = call "wait.vi"("milliseconds to wait"="preSTS delay [ms]", "application reference in"=w359) -> ("application reference out"=w381:refnum<vi>)  [unwired: 8 in, 1 out]
            n165 = call <userlib>:"BiasSpectroscopy Start.vi"("Application ref in"=w381, "Get data (F)"=TRUE ("Get Data (F)"), "Error in (no error)"=w398) -> ("Application ref out"=w371:refnum<vi>, "Data"=w397:sgl[][], "Parameters"=w396:sgl[], "Error out"=w389:errorcluster)  [unwired: 8 in, 1 out]
            n166 = local read "Move Bias"() -> (w377:dbl)
            n167 = call <userlib>:"Lockin Mod on_off Set.vi"("Lockin ON/OFF"=FALSE, "Application ref in"=w371) -> ("Application ref out"=w370:refnum<vi>)  [unwired: 8 in, 1 out]
            n168 = call "SafeBiasSet.vi"("Application ref in"=w370, "Bias (V)"=w377, "Ramp"=w360) -> ("Application ref out"=w373:refnum<vi>)  [unwired: 6 in, 1 out]
            n169 = local read "Move Current"() -> (w376:dbl)
            n170 = Delete From Array(array=w397, length=1, index (row)=0 ("index")) -> (array with subset deleted=w395:sgl[][])  [unwired: 1 in, 1 out]
            n171 = call <userlib>:"Ctrl-on_off Set.vi"("Z Controller ON/OFF"=TRUE, "Application ref in"=w373) -> ("Application ref out"=w372:refnum<vi>)  [unwired: 8 in, 1 out]
            n172 = Write to Binary File(file (use dialog)=w401, data=w396, error in=w389, 5:FALSE ("prepend array or string size? (T)")) -> (refnum out=w400:refnum<file>, error out=w388:errorcluster)  [unwired: 2 in, 1 out]
            n173 = call <userlib>:"Z-Ctrl Setpoint Set.vi"("Z Controller setpoint"=w376, "Application ref in"=w372) -> ("Application ref out"=w378:refnum<vi>)  [unwired: 8 in, 1 out]
            n174 = Increment(x=w386) -> (x+1=w385:i32)
            n175 = Write to Binary File(file (use dialog)=w400, data=w395, error in=w388, 5:FALSE ("prepend array or string size? (T)")) -> (refnum out=w399:refnum<file>, error out=w387:errorcluster)  [unwired: 2 in, 1 out]
          }
        }
        n176 = Get Date/Time In Seconds() -> (seconds since 1Jan1904=w195:timestamp)
        n177 = local read "total Points"() -> (w201:i32)
        n178 = Subtract(x=w195, y=w200) -> (x-y=w199:dbl)
        n179 = Divide(x=w198, y=w201) -> (x/y=w204:dbl)
        n180 = Subtract(x=w201, y=w198) -> (x-y=w196:i32)
        n181 = Divide(x=w199, y=w198) -> (x/y=w197:dbl)
        n182 = Multiply(x=w197, y=w196) -> (x*y=w194:dbl)
        "remaining" <- w194
        n183 = Multiply(x=w204, y=100.0) -> (x*y=→"Progress":dbl)
        n184 = Add(x=w195, y=w194) -> (x+y=→"ETA":timestamp)
      }
      frame "end" {
        n185 = Close File(refnum=w432) -> ()  [unwired: 1 in, 2 out]
        n186 = Close File(refnum=w430) -> (path=w429:path)  [unwired: 1 in, 1 out]
        n187 = local write "Status"("finishing" ("Status")) -> ()
        n188 = call "STSGrid.vi"("Binary Spectroscopy File"=w429) -> ()  [unwired: 11 in]
        n189 = Bundle(w437, w437) -> (w459:cluster{sgl[][], sgl[][]})  [unwired: 1 in]
        n190 = Build Array(w459) -> (w458:cluster{sgl[][], sgl[][]}[])
        n191 = Unbundle By Name(w447) -> ("center X (m)"=w445:sgl, "center Y (m)"=w444:sgl, "angle (deg)"=w443:sgl, "width (m)"=w442:sgl, "height (m)"=w441:sgl)
        n192 = Strip Path(path=w421) -> (stripped path=w451:path, name=w450:string)
        n193 = Get Date/Time In Seconds() -> (seconds since 1Jan1904=w417:timestamp)
        n194 = Bundle By Name(cluster=T5 {"up/down"=FALSE, "time/line"=0.0, "start time"=timestamp(0 s since 1904-01-01), "end time"=timestamp(0 s since 1904-01-01)} ("Scan param"), "up/down"=TRUE, "time/line"=sgl nan ("input 7"), "start time"=w455, "end time"=w417) -> (w454:T5)
        n195 = Bundle By Name(cluster=T3 {"center X"=0.0, "center Y"=0.0, "angle"=0.0, "width"=0.0, "height"=0.0, "# pixels"=0, "# lines"=0} ("Scanfield"), "center X"=w445, "center Y"=w444, "angle"=w443, "width"=w442, "height"=w441, "# lines"=w438, "# pixels"=w439) -> (w440:T3)
        n196 = Bundle("stripped path"=w451, "name"=w450) -> (w449:cluster{"stripped path":path, "name":string})  [unwired: 1 in]
        n197 = call <userlib>:"Save sxm File.vi"("Auto file naming? (T)"=FALSE, "Scanfield"=w440, "Scan param"=w454, "error in (no error)"=w448, "Channels data"=w458, "Channels config"=T4 [{"Name"="Z (m)", "Calibration"=1.0, "Offset"=0.0, "Channel index"=0}], "Filename control"=w449) -> ("error out"=w426:errorcluster)  [unwired: 2 in, 2 out]
        n198 = Strip Path(path=w421) -> (stripped path=w428:path)  [unwired: 1 out]
        n199 = call <userlib>:"Get Session Path.vi"("error in (no error)"=w426, "Application ref in"=w425) -> ("error out"=w422:errorcluster, "Session path"=w424:path, "Application ref out"=w405:refnum<vi>)  [unwired: 7 in]
        n200 = Path To String(path=w421) -> (string=w420:string)
        n201 = Strip Path(path=w428) -> (stripped path=w406:path)  [unwired: 1 out]
        n202 = call "SXM.vi"("Path"=w424, "Delete"=FALSE, "error in"=w422) -> ("error out"=w403:errorcluster)  [unwired: 7 in]
        n203 = call <userlib>:"Set Session Path.vi"("error in (no error)"=w403, "Session Folder"=w406, "Application ref in"=w405) -> ("error out"=w402:errorcluster, "Application ref out"=w404:refnum<vi>)  [unwired: 7 in]
        n204 = Format Date/Time String(time format string (%c)=" Finished at %y%m%d - %H%M%S ", seconds (now)=w417) -> (date/time string=w416:string)  [unwired: 1 in]
        n205 = Concatenate Strings(w420, "\r\n", w416) -> (w419:string)
        n206 = Search and Replace String(input string="Email when finished", search string="@") -> (number of replacements=w412:i32)  [unwired: 6 in, 3 out]
        n207 = Greater Than 0?(x=w412) -> (x > 0?=w411:bool)
        n208 = case shown="True" w411 {
          tunnel: w402 -> [_ w466]
          tunnel: w419 -> [_ w464]
          tunnel: "Email when finished" -> [_ w463]
          frame False {
          }
          frame True {
            n209 = call "Send Email"("error in"=w466, "Message"=w464, "Subject"="Grid Finished", "Recipients"=w463) -> ()  [unwired: 7 in, 1 out]
          }
        }
        n210 = call <userlib>:"BiasSpectroscopy SetProperties.vi"("Application ref in"=w404, "Z-Controller hold (no change)"=enum16{"no change", "on", "off"}."on") -> ("Application ref out"=w409:refnum<vi>)  [unwired: 12 in, 1 out]
        n211 = call <userlib>:"TipLift Set.vi"("TipLift (m)"=sgl 0.0, "Application ref in"=w409) -> ("Application ref out"=w408:refnum<vi>)  [unwired: 8 in, 1 out]
      }
    }
    "Error out" <- w43
    "Points taken" <- w11
    "X Offset" <- w10
    "Y Offset" <- w9
  }
